vi "Handle Player.vi"(5 "Maze (0: Empty, -1: Enemy. >0: Teammate":i32[][](array[numeric]), 7 "p":i32, 9 "Additional Wait":i32, 10 "Data":T1) -> (1 "Output":T5, 2 "Data out":T1)   [LabVIEW 2015, in "TeamEffort.lvclass"]
uses:
  TeamEffort.lvclass
  Grid Cluster.ctl
  Player Cluster.ctl
  Square/Square.lvclass
  Team Move Input.ctl
  Type Defs/Action Enum.ctl
  Team Move Output.ctl
  Type Defs/Direction Enum.ctl
  Type Defs/SB Type Defs.lvlib
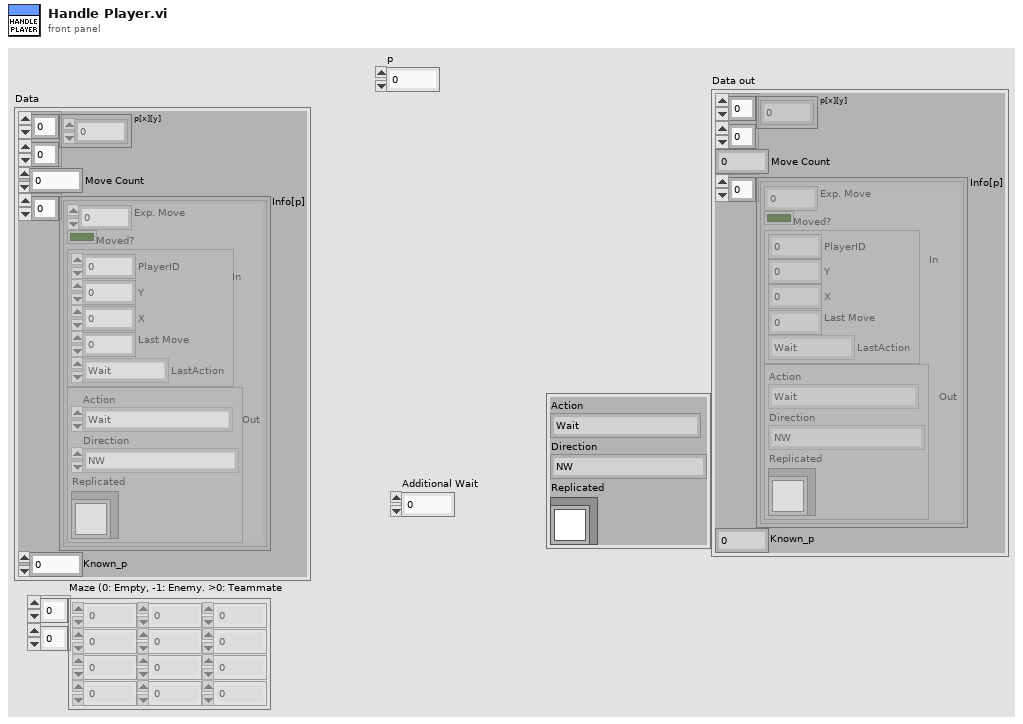
[diagram p1: front panel]
types:
  T1 = typedef "TeamEffort.lvclass/Grid Cluster.ctl" = cluster{"p[x][y]":i32[][], "Move Count":i32, "Info[p]":T2[], "Known_p":i32}
  T2 = typedef "TeamEffort.lvclass/Player Cluster.ctl" = cluster{"Exp. Move":i32, "Moved?":bool, "In":T3, "Out":T5}
  T3 = typedef "TeamEffort.lvclass/Team Move Input.ctl" = cluster{"PlayerID":i32, "Y":i32, "X":i32, "Last Move":i32, "LastAction":T4}
  T4 = typedef "SB Type Defs.lvlib/Action Enum.ctl" = enum16{"Wait", "Move", "Attack", "Replicate"}
  T5 = typedef "TeamEffort.lvclass/Team Move Output.ctl" = cluster{"Action":T4, "Direction":T6, "Replicated":refnum<class "Square.lvclass">}
  T6 = typedef "SB Type Defs.lvlib/Direction Enum.ctl" = enum16{"NW", "N", "NE", "E", "SE", "S", "SW", "W"}
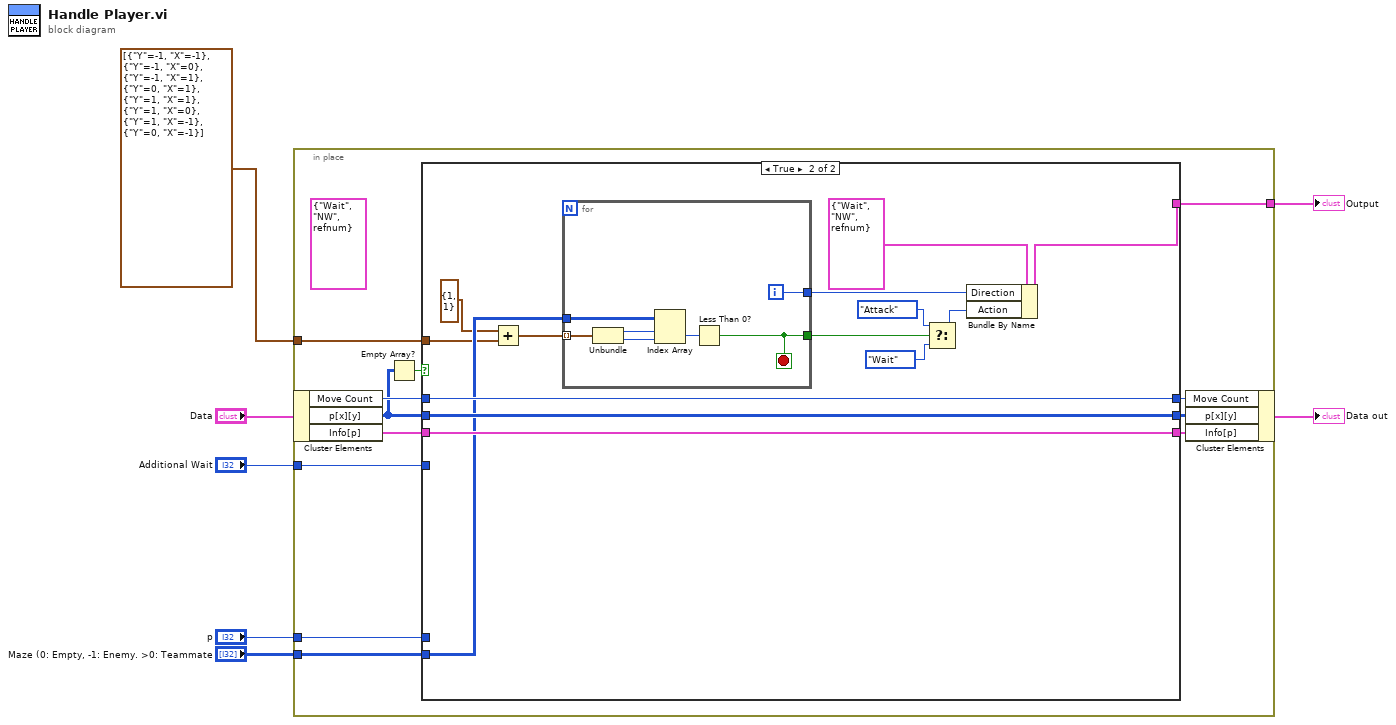
[diagram p0: block diagram]
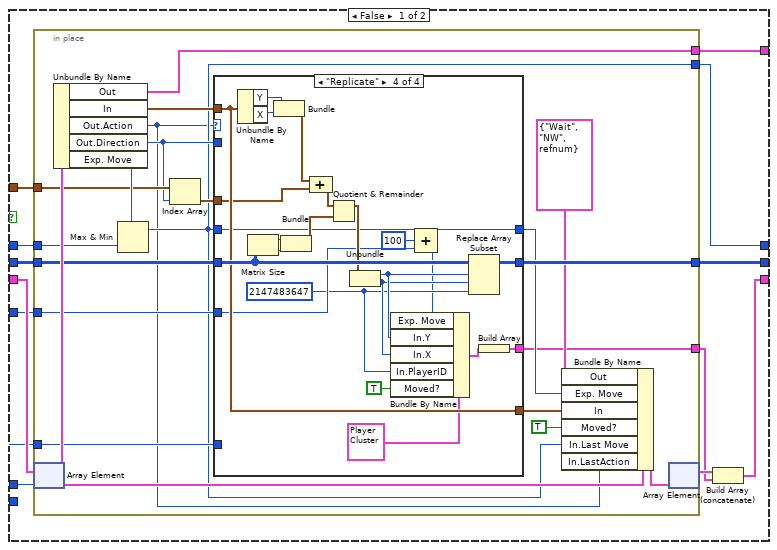
[diagram p2: hidden frame]
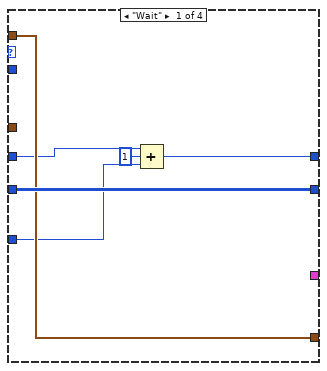
[diagram p3: hidden frame]
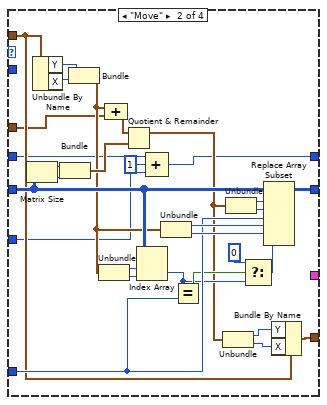
[diagram p4: hidden frame]
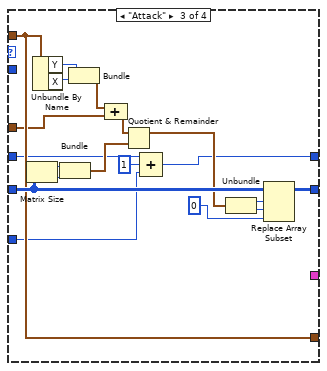
[diagram p5: hidden frame]
diagram:
  n1 = in-place {
    in-place-border: "p" -> [w14]
    in-place-border: [w17] -> w5
    in-place-border: cluster{"Y":i32, "X":i32}[] [{"Y"=-1, "X"=-1}, {"Y"=-1, "X"=0}, {"Y"=-1, "X"=1}, {"Y"=0, "X"=1}, {"Y"=1, "X"=1}, {"Y"=1, "X"=0}, {"Y"=1, "X"=-1}, {"Y"=0, "X"=-1}] -> [w13]
    in-place-border: "Additional Wait" -> [w12]
    in-place-border: "Maze (0: Empty, -1: Enemy. >0: Teammate" -> [w8]
    (unwired) T5 {"Action"=enum."Wait", "Direction"=enum."NW", "Replicated"=refnum} ("Output")
    n2 = in-place-cluster #1("Data") -> ("Move Count"=w18:i32, "p[x][y]"=w10:i32[][], "Info[p]"=w19:T2[])
    n3 = Empty Array?(array=w10) -> (empty?=w9:bool)
    n4 = case shown="True" w9 {
      tunnel: w19 -> [w31 w141]
      tunnel: w18 -> [w30 w142]
      tunnel: [w29 w135] -> w17
      tunnel: [w28 w142] -> w16
      tunnel: [w26 w143] -> w15
      tunnel: w14 -> [w25 _]
      tunnel: w13 -> [w24 w138]
      tunnel: w12 -> [w23 _]
      tunnel: [w22 w141] -> w11
      tunnel: w10 -> [w20 w143]
      tunnel: w8 -> [_ w140]
      frame False {
        n5 = in-place {
          in-place-border: w30 -> [w47]
          in-place-border: [w33] -> w28
          in-place-border: w20 -> [w46]
          in-place-border: [w45] -> w26
          in-place-border: [w42] -> w29
          in-place-border: w25 -> [w40]
          in-place-border: w24 -> [w39]
          in-place-border: w23 -> [w36]
          in-place-border: [w34] -> w21
          n6 = in-place-array #2(w31, w25) -> (w49:T2)
          n7 = Unbundle By Name(w49) -> ("Out"=w42:T5, "In"=w41:T3, "Out.Action"=w32:T4, "Out.Direction"=w38:T6, "Exp. Move"=w48:i32)
          n8 = Max & Min(x=w48, y=w47) -> (max(x,y)=w33:i32)  [unwired: 1 out]
          n9 = Index Array(array=w39, index=w38) -> (element=w37:cluster{"Y":i32, "X":i32})
          n10 = case shown="\"Replicate\"" w32 {
            tunnel: w46 -> [w57 w87 w106 w129]
            tunnel: [w57 w80 w99 w122] -> w45
            tunnel: w33 -> [w55 w61 w91 w117]
            tunnel: [w52 w59 w90 w107] -> w43
            tunnel: [w56 w65 w93 w120] -> w44
            tunnel: w41 -> [w56 w66 w93 w120]
            tunnel: w38 -> [_ _ _ _]
            tunnel: w40 -> [_ w70 _ _]
            tunnel: w37 -> [_ w62 w92 w118]
            tunnel: w36 -> [w54 w60 w89 w115]
            tunnel: [_ _ _ w108] -> w34
            frame "Wait" {
              n11 = Compound Arithmetic op=ADD(w55, 1 ("value"), w54) -> (w52:i32)
            }
            frame "Move" {
              n12 = Matrix Size(0:w87) -> (1:w86:i32, 2:w85:i32)
              n13 = Unbundle By Name(w66) -> ("Y"=w83:i32, "X"=w84:i32)
              n14 = Bundle("number of columns"=w86, "matrix"=w85) -> (w81:cluster{"number of columns":i32, "matrix":i32})  [unwired: 1 in]
              n15 = Bundle("Y"=w83, "X"=w84) -> (w75:cluster{"Y":i32, "X":i32})  [unwired: 1 in]
              n16 = Unbundle(w75) -> ("Y"=w77:i32, "X"=w76:i32)
              n17 = Compound Arithmetic op=ADD(w75, w62) -> (w82:cluster{"Y":i32, "X":i32})
              n18 = Quotient & Remainder(x=w82, y=w81) -> (x-y*floor(x/y)=w67:cluster{i32, i32})  [unwired: 1 out]
              n19 = Index Array(array=w87, index (row)=w77, index (col)=w76) -> (element=w68:i32)
              n20 = Compound Arithmetic op=ADD(w61, 1 ("value"), w60) -> (w59:i32)
              n21 = Unbundle(w75) -> ("Y"=w74:i32, "X"=w73:i32)
              n22 = Equal?(x=w68, y=w70) -> (x = y?=w69:bool)
              n23 = Unbundle(w67) -> (w64:i32, w63:i32)
              n24 = Unbundle(w67) -> (w79:i32, w78:i32)
              n25 = Select(t=0, s=w69, f=w68) -> (s? t:f=w72:i32)
              n26 = Replace Array Subset(array=w87, new element #1=w70, index (row) #1=w79, index (col) #1=w78, new element #2=w72, index (row) #2=w74, index (col) #2=w73) -> (w80:i32[][])
              n27 = Bundle By Name(cluster=w66, "Y"=w64, "X"=w63) -> (w65:T3)
            }
            frame "Attack" {
              n28 = Matrix Size(0:w106) -> (1:w105:i32, 2:w104:i32)
              n29 = Unbundle By Name(w93) -> ("Y"=w102:i32, "X"=w103:i32)
              n30 = Bundle("number of columns"=w105, "matrix"=w104) -> (w100:cluster{"number of columns":i32, "matrix":i32})  [unwired: 1 in]
              n31 = Bundle("Y"=w102, "X"=w103) -> (w96:cluster{"Y":i32, "X":i32})  [unwired: 1 in]
              n32 = Compound Arithmetic op=ADD(w96, w92) -> (w101:cluster{"Y":i32, "X":i32})
              n33 = Quotient & Remainder(x=w101, y=w100) -> (x-y*floor(x/y)=w95:cluster{i32, i32})  [unwired: 1 out]
              n34 = Compound Arithmetic op=ADD(w91, 1 ("value"), w89) -> (w90:i32)
              n35 = Unbundle(w95) -> (w98:i32, w97:i32)
              n36 = Replace Array Subset(array=w106, new element=0 ("new element/subarray"), index (row)=w98, index (col)=w97) -> (w99:i32[][])
            }
            frame "Replicate" {
              w112 = 2147483647 ("new element/subarray")
              n37 = Unbundle By Name(w120) -> ("Y"=w125:i32, "X"=w126:i32)
              n38 = Matrix Size(0:w129) -> (1:w128:i32, 2:w127:i32)
              n39 = Bundle("Y"=w125, "X"=w126) -> (w121:cluster{"Y":i32, "X":i32})  [unwired: 1 in]
              n40 = Bundle("number of columns"=w128, "matrix"=w127) -> (w123:cluster{"number of columns":i32, "matrix":i32})  [unwired: 1 in]
              n41 = Compound Arithmetic op=ADD(w121, w118) -> (w124:cluster{"Y":i32, "X":i32})
              n42 = Quotient & Remainder(x=w124, y=w123) -> (x-y*floor(x/y)=w119:cluster{i32, i32})  [unwired: 1 out]
              n43 = Unbundle(w119) -> (w114:i32, w113:i32)
              n44 = Compound Arithmetic op=ADD(w117, 100 ("value"), w115) -> (w107:i32)
              n45 = Bundle By Name(cluster=T2 {"Exp. Move"=0, "Moved?"=FALSE, "In"={"PlayerID"=0, "Y"=0, "X"=0, "Last Move"=0, "LastAction"=enum."Wait"}, "Out"={"Action"=enum."Wait", "Direction"=enum."NW", "Replicated"=refnum}} ("element"), "Exp. Move"=w107, "In.Y"=w114, "In.X"=w113, "In.PlayerID"=w112, "Moved?"=TRUE) -> (w109:T2)
              n46 = Replace Array Subset(array=w129, new element=w112, index (row)=w114, index (col)=w113) -> (w122:i32[][])
              n47 = Build Array(w109) -> (w108:T2[])
            }
          }
          n48 = Bundle By Name(cluster=w49, "Out"=T5 {"Action"=enum."Wait", "Direction"=enum."NW", "Replicated"=refnum}, "Exp. Move"=w43, "In"=w44, "Moved?"=TRUE, "In.Last Move"=w33, "In.LastAction"=w32) -> (w50:T2)
          n49 = in-place-array #2(w50) -> (w27:T2[])  [unwired: 1 out]
        }
        n50 = Build Array (concatenate)(w27, w21) -> (w22:T2[])
      }
      frame True {
        n51 = Add(x=cluster{"Y":i32, "X":i32} {"Y"=1, "X"=1}, y=w138) -> (x+y=w137:cluster{"Y":i32, "X":i32}[])
        n52 = for {
          tunnel: w140 -> [w150]
          tunnel: w137 -> [w149] mode=indexing
          tunnel: [w145] -> w133
          tunnel: [w144] -> w134
          i -> [w144]
          stop <- w145 stop-if-true
          n53 = Unbundle(w149) -> ("Y"=w148:i32, "X"=w147:i32)
          n54 = Index Array(array=w150, index (row)=w148, index (col)=w147) -> (element=w146:i32)
          n55 = Less Than 0?(x=w146) -> (x < 0?=w145:bool)
        }
        n56 = Select(t=Action_Enum."Attack" ("Action"), s=w133, f=Action_Enum."Wait" ("Action")) -> (s? t:f=w130:T4)
        n57 = Bundle By Name(cluster=T5 {"Action"=enum."Wait", "Direction"=enum."NW", "Replicated"=refnum} ("Out"), "Direction"=w134, "Action"=w130) -> (w135:T5)
      }
    }
    n58 = in-place-cluster #1("Move Count"=w16, "p[x][y]"=w15, "Info[p]"=w11) -> (→"Data out":T1)
  }
  "Output" <- w5
